vi "Handle Messages.vi"(8 "error in (no error)":errorcluster, 9 "Message Data":variant, 10 "Message":string, 11 "Mock Rig Process In":refnum<class "Mock Process.lvclass">) -> (0 "error out":errorcluster, 3 "Mock Rig Process Out":refnum<class "Mock Process.lvclass">)   [LabVIEW 2020, in "Mock Process.lvclass"]
uses:
  Mock Process.lvclass
  C:/Users/anton/Documents/GitHub/Triarc-Framework/source/Framework/Helper Loop/Helper Loop.lvclass
  Mock Process.lvclass/Mock Process.ctl
  Framework/Process/Process.lvclass
  Framework/Helper Loop/Helper Loop.lvclass
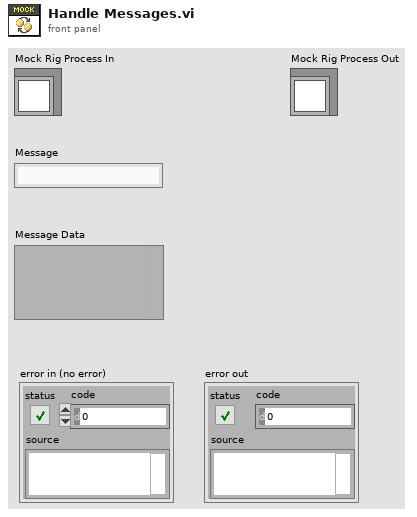
[diagram p1: front panel]
types:
  T1 = cluster{"Message":string, "Message Data":variant}
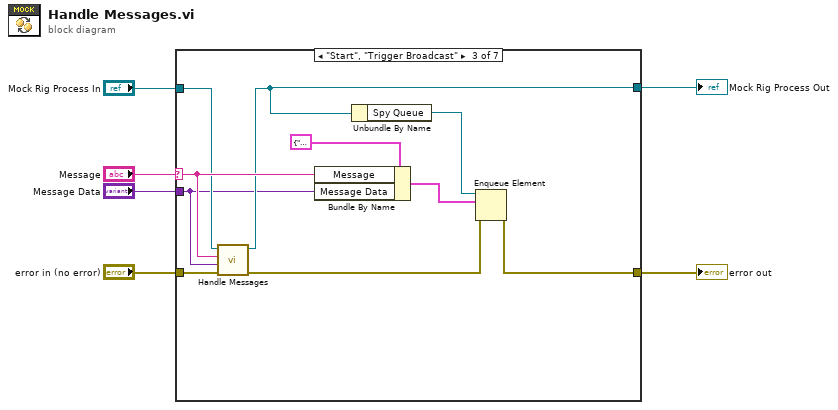
[diagram p0: block diagram]
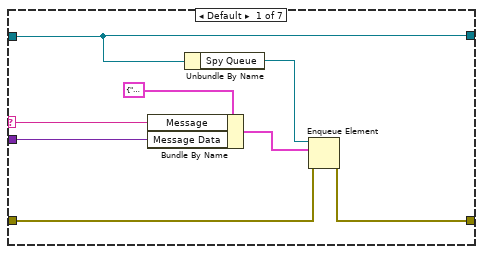
[diagram p2: hidden frame]
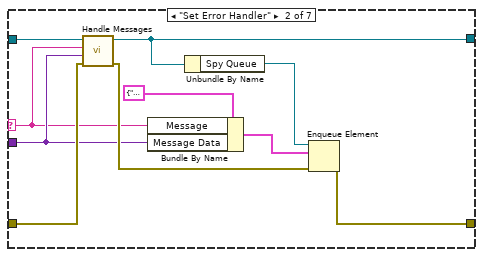
[diagram p3: hidden frame]
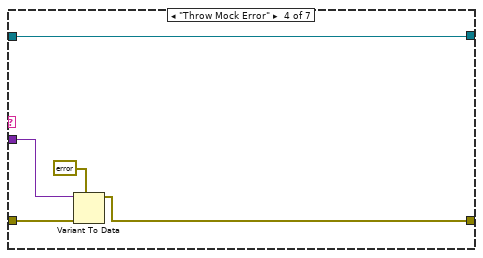
[diagram p4: hidden frame]
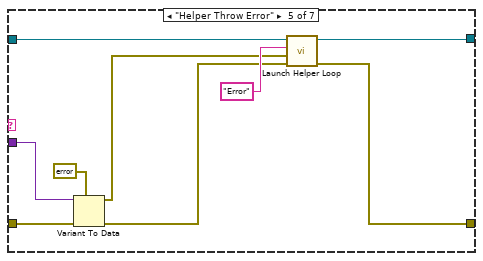
[diagram p5: hidden frame]
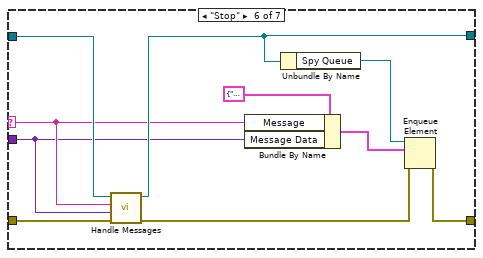
[diagram p6: hidden frame]
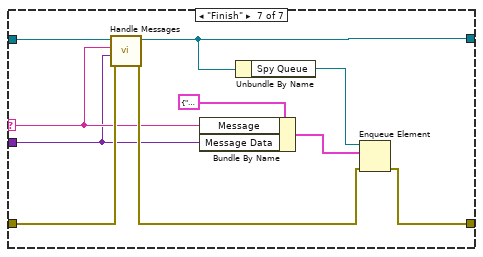
[diagram p7: hidden frame]
diagram:
  n1 = case shown="\"Start\", \"Trigger Broadcast\"" "Message" {
    selector: "Message" -> [w10 w15 w28 _ _ w50 w60]
    tunnel: [w8 w20 w30 w35 w40 w55 w61] -> w6
    tunnel: [w7 w17 w27 w39 w44 w52 w63] -> w5
    tunnel: "error in (no error)" -> [w9 w21 w31 w38 w48 w53 w67]
    tunnel: "Message Data" -> [w11 w16 w25 w37 w47 w49 w59]
    tunnel: "Mock Rig Process In" -> [w7 w18 w26 w39 w43 w51 w68]
    frame Default {
      n2 = Bundle By Name(cluster=T1 {"Message"="", "Message Data"=variant} ("Message Cluster"), "Message"=w10, "Message Data"=w11) -> (w14:T1)
      n3 = Unbundle By Name(w7) -> ("Spy Queue"=w12:refnum<queue>)
      n4 = Enqueue Element(queue=w12, element=w14, error in (no error)=w9) -> (error out=w8:errorcluster)  [unwired: 1 in, 2 out]
    }
    frame "Set Error Handler" {
      n5 = call-parent "Handle Messages.vi"("error in (no error)"=w21, "Message Data"=w16, "Message"=w15, "Process In"=w18) -> ("error out"=w19:errorcluster, "Process Out"=w17:refnum<class "Mock Process.lvclass">)  [unwired: 6 in]
      n6 = Bundle By Name(cluster=T1 {"Message"="", "Message Data"=variant} ("Message Cluster"), "Message"=w15, "Message Data"=w16) -> (w24:T1)
      n7 = Unbundle By Name(w17) -> ("Spy Queue"=w22:refnum<queue>)
      n8 = Enqueue Element(queue=w22, element=w24, error in (no error)=w19) -> (error out=w20:errorcluster)  [unwired: 1 in, 2 out]
    }
    frame "Start", "Trigger Broadcast" {
      n9 = call-parent "Handle Messages.vi"("error in (no error)"=w31, "Message Data"=w25, "Message"=w28, "Process In"=w26) -> ("error out"=w29:errorcluster, "Process Out"=w27:refnum<class "Mock Process.lvclass">)  [unwired: 6 in]
      n10 = Bundle By Name(cluster=T1 {"Message"="", "Message Data"=variant} ("Message Cluster"), "Message"=w28, "Message Data"=w25) -> (w34:T1)
      n11 = Unbundle By Name(w27) -> ("Spy Queue"=w32:refnum<queue>)
      n12 = Enqueue Element(queue=w32, element=w34, error in (no error)=w29) -> (error out=w30:errorcluster)  [unwired: 1 in, 2 out]
    }
    frame "Throw Mock Error" {
      n13 = Variant To Data(error in=w38, type=errorcluster {"status"=FALSE, "code"=0, "source"=""} ("error out"), Variant=w37) -> (data=w35:errorcluster)  [unwired: 1 out]
    }
    frame "Helper Throw Error" {
      n14 = Variant To Data(error in=w48, type=errorcluster {"status"=FALSE, "code"=0, "source"=""} ("error out"), Variant=w47) -> (data=w41:errorcluster, error out=w42:errorcluster)
      n15 = call "Launch Helper Loop.vi"("error in (no error)"=w42, "Message Data"=w41, "Message"="Error", "Helper Loop In"=w43) -> ("error out"=w40:errorcluster, "Helper Loop Out"=w44:refnum<class "Mock Process.lvclass">)  [unwired: 6 in]
    }
    frame "Stop" {
      n16 = call-parent "Handle Messages.vi"("error in (no error)"=w53, "Message Data"=w49, "Message"=w50, "Process In"=w51) -> ("error out"=w54:errorcluster, "Process Out"=w52:refnum<class "Mock Process.lvclass">)  [unwired: 6 in]
      n17 = Bundle By Name(cluster=T1 {"Message"="", "Message Data"=variant} ("Message Cluster"), "Message"=w50, "Message Data"=w49) -> (w58:T1)
      n18 = Unbundle By Name(w52) -> ("Spy Queue"=w56:refnum<queue>)
      n19 = Enqueue Element(queue=w56, element=w58, error in (no error)=w54) -> (error out=w55:errorcluster)  [unwired: 1 in, 2 out]
    }
    frame "Finish" {
      n20 = call-parent "Handle Messages.vi"("error in (no error)"=w67, "Message Data"=w59, "Message"=w60, "Process In"=w68) -> ("error out"=w62:errorcluster, "Process Out"=w63:refnum<class "Mock Process.lvclass">)  [unwired: 6 in]
      n21 = Bundle By Name(cluster=T1 {"Message"="", "Message Data"=variant} ("Message Cluster"), "Message"=w60, "Message Data"=w59) -> (w66:T1)
      n22 = Unbundle By Name(w63) -> ("Spy Queue"=w65:refnum<queue>)
      n23 = Enqueue Element(queue=w65, element=w66, error in (no error)=w62) -> (error out=w61:errorcluster)  [unwired: 1 in, 2 out]
    }
  }
  "error out" <- w6
  "Mock Rig Process Out" <- w5
